vi "post_operator.vi"(8 "error in (no error)":errorcluster, 10 "Small?":bool, 11 "operator":T1 {"Operator" items=["Giraffe", "Andrew Collette", "Keith Drake", "Anthony Shu", "Evan Thomas", "Nicholaus Beaty", "David James", "John Fontanese", "Bill Goode", "Zach Ulibarri", ""]}) -> (0 "error out":errorcluster)   [LabVIEW 2015]
doc: "Adds a new row to the dcs_spot table."
uses:
  User Interface/Controls/Operator.ctl
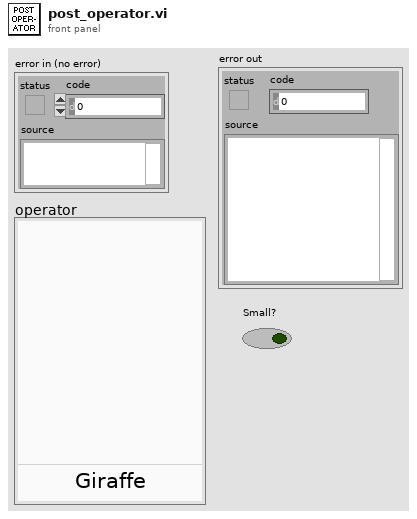
[diagram p1: front panel]
types:
  T1 = typedef "Operator.ctl" = cluster{"Timestamp":i64, "Operator":u16}
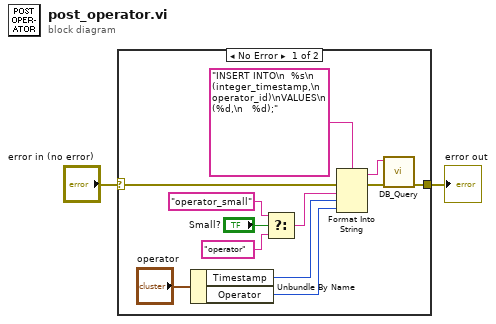
[diagram p0: block diagram]
diagram:
  n1 = case shown="No Error" "error in (no error)" {
    selector: "error in (no error)" -> [w14 w15]
    tunnel: [w8 w15] -> w1
    frame No Error {
      n2 = Unbundle By Name("operator") -> ("Timestamp"=w11:i64, "Operator"=w10:u16)
      n3 = Select(t="operator_small" ("Parameterized Query"), s="Small?", f="operator" ("Parameterized Query")) -> (s? t:f=w4:string)
      n4 = Format Into String(format string="INSERT INTO\n  %s\n  (integer_timestamp,\n   operator_id)\nVALUES\n  (%d,\n   %d);" ("Parameterized Query"), error in=w14, w4, w11, w10) -> (resulting string=w9:string, error out=w13:errorcluster)  [unwired: 1 in]
      n5 = call "DB_Query.vi"("error in (no error)"=w13, "Parameterized Query"=w9) -> ("error out"=w8:errorcluster)  [unwired: 7 in, 2 out]
    }
    frame Error {
    }
  }
  "error out" <- w1
